vi "GerenateKey.vi"(1 "Array":i32[](array[numeric])) -> (0 "Numeric":i32)   [LabVIEW 2016]
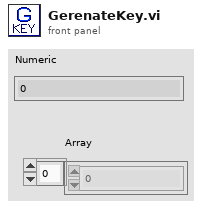
[diagram p1: front panel]
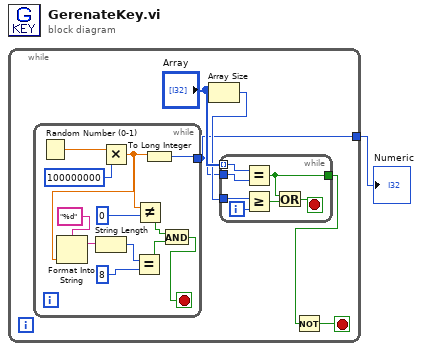
[diagram p0: block diagram]
diagram:
  n1 = while {
    tunnel: [w4] -> w1
    stop <- w3 stop-if-true
    n2 = while {
      tunnel: [w14] -> w4
      stop <- w17 stop-if-true
      n3 = Random Number (0-1)() -> (number: 0 to 1=w24:dbl)
      n4 = Multiply(x=w24, y=100000000) -> (x*y=w15:dbl)
      n5 = Format Into String(format string="%d", w15) -> (resulting string=w23:string)  [unwired: 2 in, 1 out]
      n6 = String Length(string=w23) -> (length=w16:i32)
      n7 = Equal?(x=w16, y=8) -> (x = y?=w18:bool)
      n8 = Not Equal?(x=w15, y=0) -> (x != y?=w19:bool)
      n9 = To Long Integer(number=w15) -> (32bit integer=w14:i32)
      n10 = And(x=w19, y=w18) -> (x .and. y?=w17:bool)
    }
    n11 = Array Size(array="Array") -> (size(s)=w5:i32)
    n12 = while {
      tunnel: "Array" -> [w11] mode=indexing
      tunnel: w4 -> [w10]
      tunnel: w5 -> [w12]
      tunnel: [w7] -> w2
      i -> [w13]
      stop <- w8 stop-if-true
      n13 = Equal?(x=w11, y=w10) -> (x = y?=w7:bool)
      n14 = Greater Or Equal?(x=w12, y=w13) -> (x >= y?=w9:bool)
      n15 = Or(x=w7, y=w9) -> (x .or. y?=w8:bool)
    }
    n16 = Not(x=w2) -> (.not. x?=w3:bool)
  }
  "Numeric" <- w1
